vi "lissajous.vi"() -> ()   [LabVIEW 2022 SP3]
panel:
  out "XY Graph 2":cluster{"Y":dbl[], "Y":dbl[]}[](graph)
  out "XY Graph":cluster{"Y":dbl[], "Y":dbl[]}[](graph)
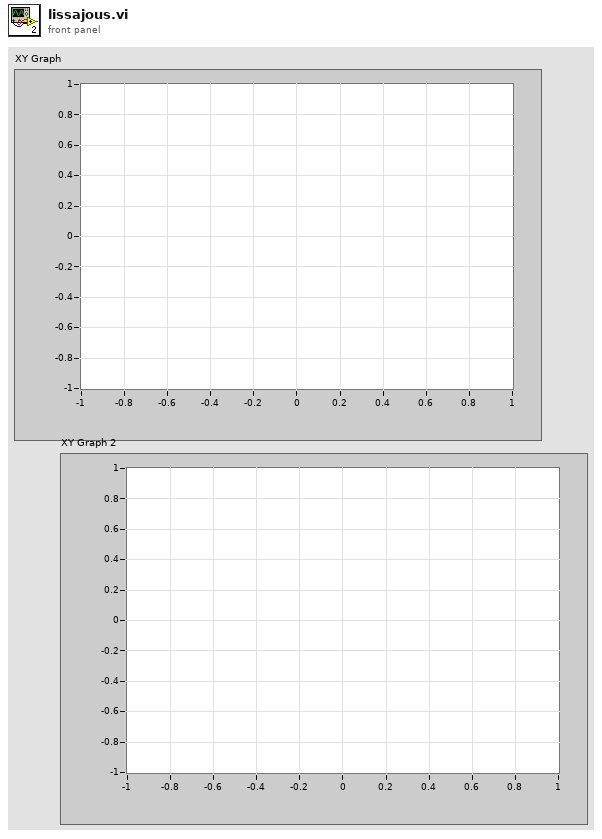
[diagram p1: front panel]
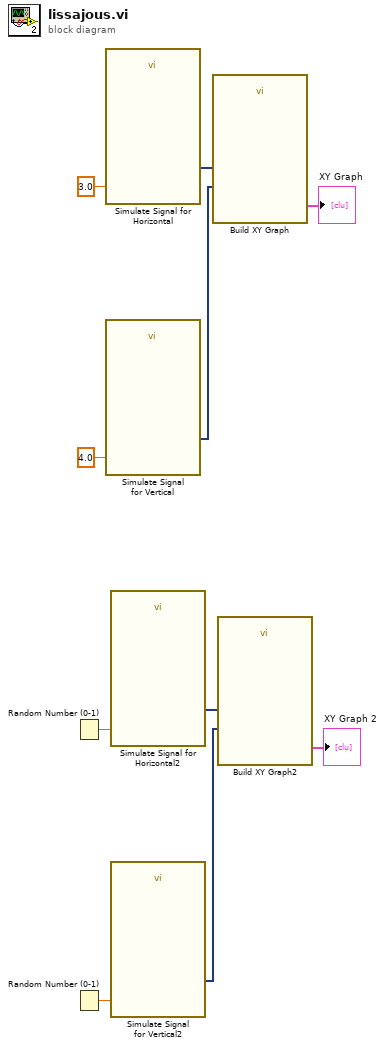
[diagram p0: block diagram]
diagram:
  n1 = Random Number (0-1)() -> (number: 0 to 1=w2:dbl)
  n2 = Random Number (0-1)() -> (number: 0 to 1=w1:dbl)
  n3 = call "Simulate Signal for Horizontal"("Frequency"=3.0) -> ("Sine"=w8:dynamicdata)  [unwired: 5 in, 9 out]
  n4 = call "Simulate Signal\nfor Vertical"("Frequency"=4.0) -> ("Sine"=w9:dynamicdata)  [unwired: 5 in, 9 out]
  n5 = call "Simulate Signal for Horizontal2"("Frequency"=w2) -> ("Sine"=w3:dynamicdata)  [unwired: 5 in, 9 out]
  n6 = call "Simulate Signal\nfor Vertical2"("Frequency"=w1) -> ("Sine"=w4:dynamicdata)  [unwired: 5 in, 9 out]
  n7 = call "Build XY Graph"("Y Input"=w9, "X Input"=w8) -> ("XY Graph"=→"XY Graph":cluster{"Y":dbl[], "Y":dbl[]}[])  [unwired: 3 in, 6 out]
  n8 = call "Build XY Graph2"("Y Input"=w4, "X Input"=w3) -> ("XY Graph"=→"XY Graph 2":cluster{"Y":dbl[], "Y":dbl[]}[])  [unwired: 3 in, 6 out]
